vi "Frames to AVI.vi"(0 "Image directory":path=path "C:/Test images", 1 "AVI output path":path=path "C:/Test.avi", 2 "Frames Per Second":u32=1, 3 "Quality":i32=1000, 4 "Format qualifier":string="*.png") -> (5 "Images used":string[](array[string]))   [LabVIEW 2014]
panel:
  out "Image":T1(plugin-control)
  out "Error Out":errorcluster
  in  "Codec":string="Microsoft Video 1"
  # "PN 10/12/2014"
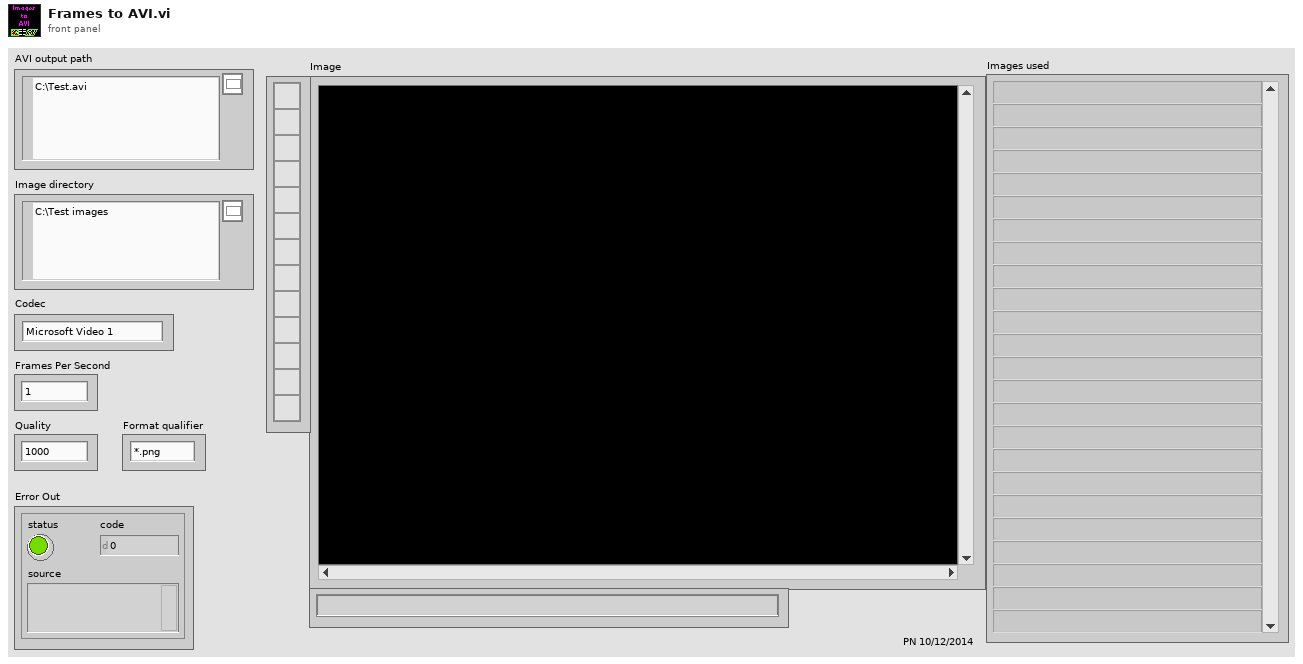
[diagram p1: front panel]
types:
  T1 = typedef "IMAQ Image.ctl" = refnum<image>
  T2 = typedef "IMAQ AVI2 Refnum.ctl" = refnum<k20>
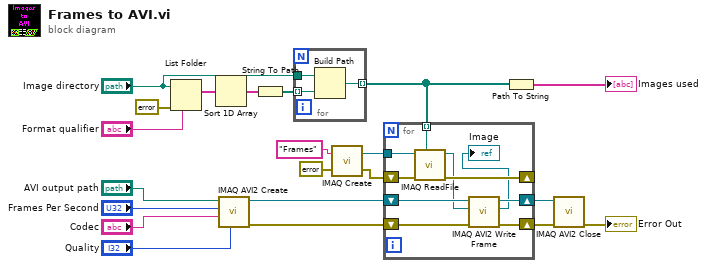
[diagram p0: block diagram]
diagram:
  n1 = List Folder(path="Image directory", pattern="Format qualifier", error in=errorcluster {"status"=FALSE, "code"=0, "source"=""}) -> (filenames=w2:string[])  [unwired: 1 in, 3 out]
  n2 = Sort 1D Array(array=w2) -> (sorted array=w1:string[])
  n3 = call "IMAQ AVI2 Create"("Quality"="Quality", "Codec"="Codec", "Frames Per Second"="Frames Per Second", "AVI Path"="AVI output path") -> ("error out"=w17:errorcluster, "AVI Refnum"=w14:T2)  [unwired: 6 in]
  n4 = String To Path(string=w1) -> (path=w11:path[])
  n5 = for {
    tunnel: w11 -> [w24] mode=indexing
    tunnel: "Image directory" -> [w23]
    tunnel: [w22] -> w5 mode=indexing
    n6 = Build Path(base path=w23, name or relative path=w24) -> (appended path=w22:path)
  }
  n7 = call "IMAQ Create"("Image Name"="Frames", "error in (no error)"=errorcluster {"status"=FALSE, "code"=0, "source"=""}) -> ("New Image"=w8:T1, "error out"=w9:errorcluster)  [unwired: 3 in]
  n8 = for {
    shift-right: [w33] -> w16
    shift-left: w17 -> [w34]
    shift-right: [w32] -> w15
    shift-left: w14 -> [w28]
    shift-right: [w30] -> _
    shift-left: w9 -> [w31]
    tunnel: w5 -> [w29] mode=indexing
    tunnel: w8 -> [w26]
    n9 = call "IMAQ ReadFile"("File Path"=w29, "error in (no error)"=w31, "Image"=w26) -> ("error out"=w30:errorcluster, "Image Out"=w27:T1)  [unwired: 4 in, 3 out]
    n10 = call "IMAQ AVI2 Write Frame"("error in (no error)"=w34, "Image"=w27, "AVI Refnum"=w28) -> ("error out"=w33:errorcluster, "Image Out (duplicate)"=→"Image":T1, "AVI Refnum (duplicate)"=w32:T2)  [unwired: 6 in]
  }
  n11 = Path To String(path=w5) -> (string=→"Images used":string[])
  n12 = call "IMAQ AVI2 Close"("error in (no error)"=w16, "AVI Refnum"=w15) -> ("error out"=→"Error Out":errorcluster)  [unwired: 9 in]
